vi "CLD 16 state machine front panel.vi"() -> ()   [LabVIEW 2019]
doc: "CLD 16 Exercise"
uses:
  CLD 16 Control Panel.ctl
  CLD 16 Status Panel.ctl
  CLD 16 state enum.ctl
panel:
  out "error out":errorcluster
  in  "error in (no error)":errorcluster
  in  "Stop Button":bool
  out "Line Two Active":bool
  out "Line One Active":bool
  in  "Control Panel Two":T1 {"Tons of Peanuts" scale=0.0..10.0}
  out "Process Control":T2 {"Process Value" format="%#.3g"}
  in  "Control Panel One":T1 {"Tons of Peanuts" scale=0.0..10.0}
  # "Display Panel"
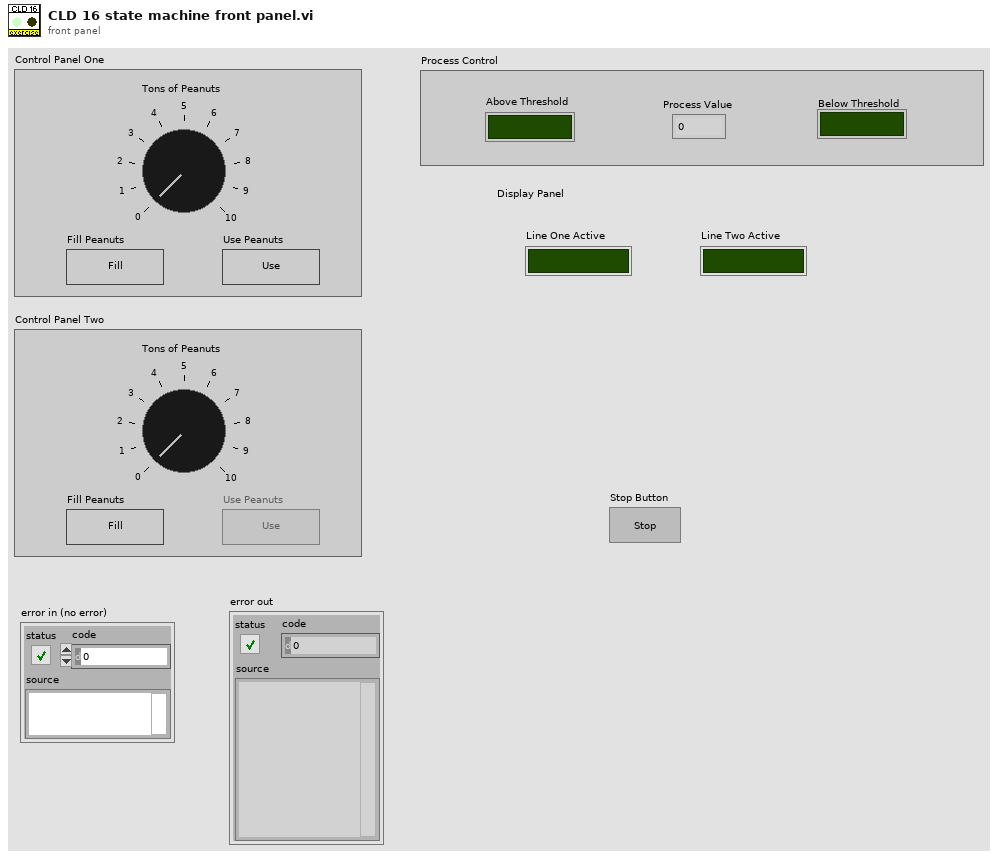
[diagram p1: front panel]
types:
  T1 = typedef "CLD 16 Control Panel.ctl" = cluster{"Tons of Peanuts":i8, "Fill Peanuts":bool, "Use Peanuts":bool}
  T2 = typedef "CLD 16 Status Panel.ctl" = cluster{"Above Threshold":bool, "Below Threshold":bool, "Process Value":dbl}
  T3 = typedef "CLD 16 state enum.ctl" = enum16{"initialize", "use", "idle"}
  T4 = enum8{"Enabled", "Disabled", "Disabled and Grayed Out"}
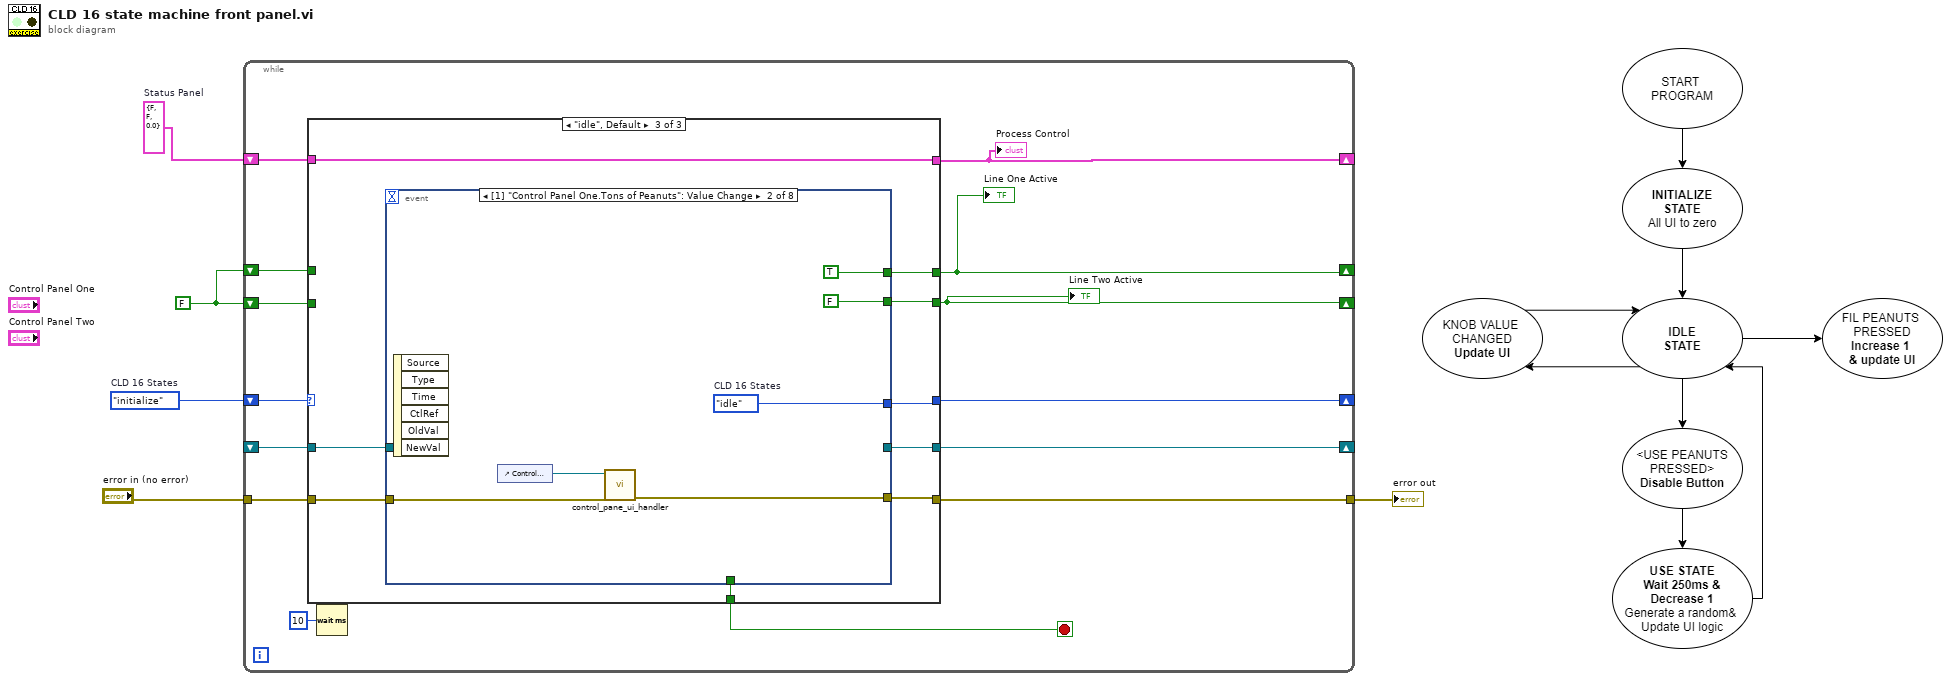
[diagram p0: block diagram]
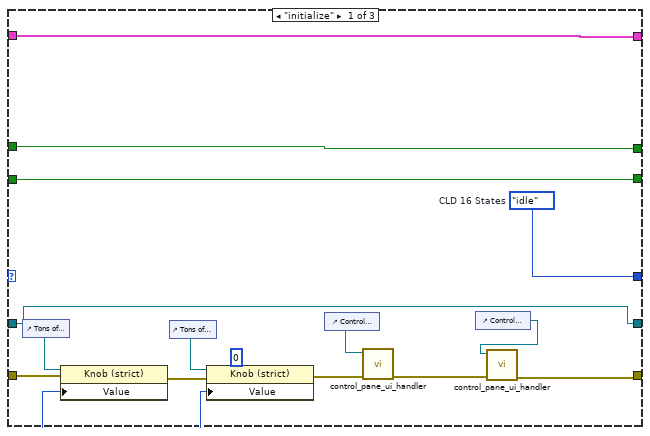
[diagram p2: hidden frame]
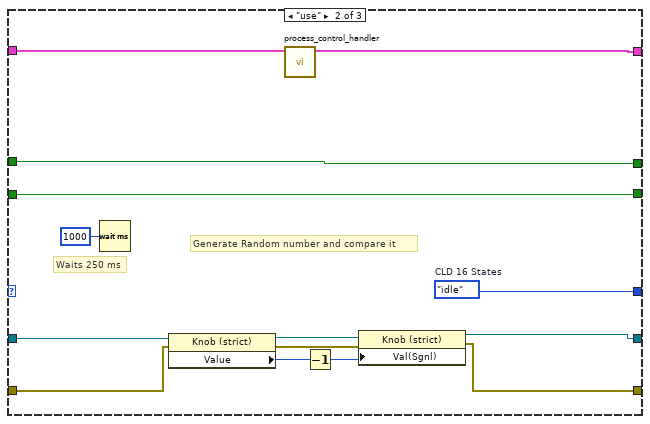
[diagram p3: hidden frame]
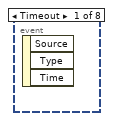
[diagram p4: hidden frame]
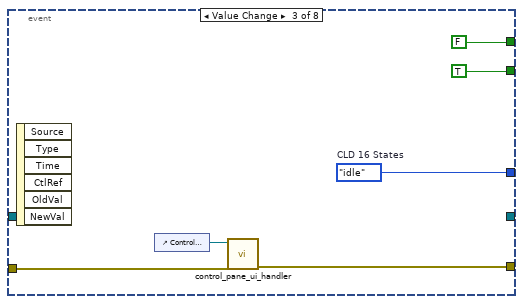
[diagram p5: hidden frame]
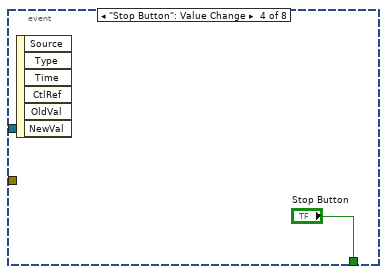
[diagram p6: hidden frame]
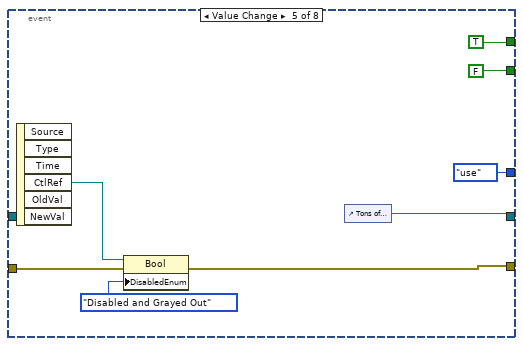
[diagram p7: hidden frame]
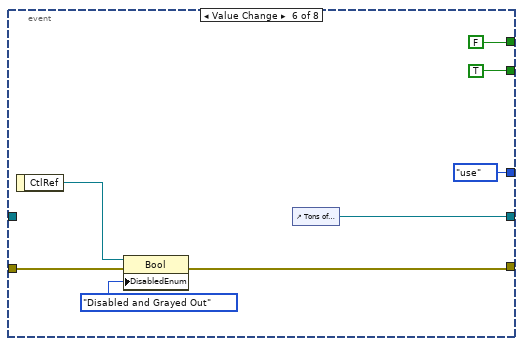
[diagram p8: hidden frame]
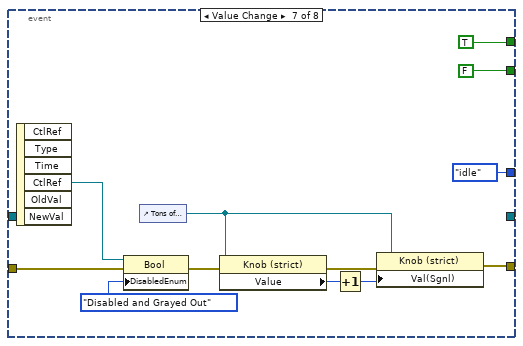
[diagram p9: hidden frame]
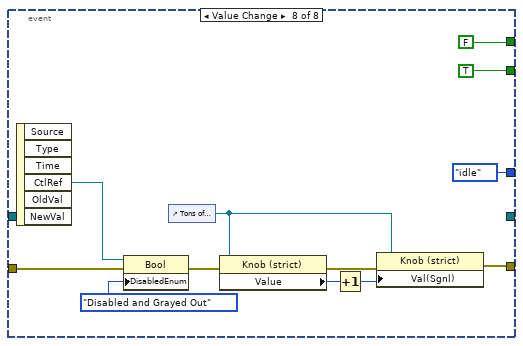
[diagram p10: hidden frame]
diagram:
  w1 = FALSE ("Line Two Active")
  w2 = T2 {"Above Threshold"=FALSE, "Below Threshold"=FALSE, "Process Value"=0.0}  # Status Panel
  w5 = CLD_16_state_enum."initialize"  # CLD 16 States
  n1 = while {
    shift-right: [w18] -> _
    shift-left: w5 -> [w19]
    tunnel: "error in (no error)" -> [w17]
    tunnel: [w16] -> w3
    shift-right: [w14] -> _
    shift-left: w2 -> [w13]
    shift-right: [w9] -> _
    shift-left: w1 -> [w12]
    shift-right: [w10] -> _
    shift-left: w1 -> [w11]
    shift-right: [w8] -> _
    shift-left: _ -> [w7]
    stop <- w6 stop-if-true
    n2 = case shown="\"idle\", Default" w19 {
      tunnel: [w23 w36 w54] -> w14
      tunnel: [w34 w48 w55] -> w18
      tunnel: w17 -> [w31 w44 w57]
      tunnel: [w25 w38 w56] -> w16
      tunnel: w13 -> [w23 w37 w54]
      tunnel: [w22 w46 w53] -> w9
      tunnel: w12 -> [w22 w46 _]
      tunnel: [w21 w45 w52] -> w10
      tunnel: w11 -> [w21 w45 _]
      tunnel: [w20 w35 w51] -> w8
      tunnel: w7 -> [w20 w43 w50]
      tunnel: [_ _ w49] -> w6
      frame "initialize" {
        w29 = i8 0 ("Value")
        w34 = CLD_16_state_enum."idle"  # CLD 16 States
        n3 = control-ref of="Tons of Peanuts"() -> (w32:refnum<vi>)
        n4 = property class="Knob (strict)"(reference=w32, error in=w31, "Value"=w29) -> (error out=w30:errorcluster)  [unwired: 1 out]
        n5 = control-ref of="Tons of Peanuts"() -> (w33:refnum<vi>)
        n6 = property class="Knob (strict)"(reference=w33, error in=w30, "Value"=w29) -> (error out=w27:errorcluster)  [unwired: 1 out]
        n7 = control-ref of="Control Panel One"() -> (w28:refnum<vi>)
        n8 = call "control_pane_ui_handler.vi"("error in (no error)"=w27, "Control Panel In"=w28) -> ("error out"=w26:errorcluster)  [unwired: 9 in]
        n9 = control-ref of="Control Panel Two"() -> (w24:refnum<vi>)
        n10 = call "control_pane_ui_handler.vi"("error in (no error)"=w26, "Control Panel In"=w24) -> ("error out"=w25:errorcluster)  [unwired: 9 in]
      }
      frame "use" {
        w48 = CLD_16_state_enum."idle"  # CLD 16 States
        # "Generate Random number and compare it"
        # "Waits 250 ms"
        n11 = Wait (ms)(milliseconds to wait=u32 1000) -> ()  [unwired: 1 out]
        n12 = property class="Knob (strict)"(reference=w43, error in=w44) -> (reference out=w42:refnum<vi>, error out=w41:errorcluster, "Value"=w40:i8)
        n13 = call "process_control_handler.vi"("Status Panel in"=w37) -> ("Status Panel out"=w36:T2)  [unwired: 10 in]
        n14 = Decrement(x=w40) -> (x-1=w39:i8)
        n15 = property class="Knob (strict)"(reference=w42, error in=w41, "Val(Sgnl)"=w39) -> (reference out=w35:refnum<vi>, error out=w38:errorcluster)
      }
      frame "idle", Default {
        n16 = event shown="[1] \"Control Panel One.Tons of Peanuts\": Value Change" {
          selector: _ -> [_ _ _ _ _ _ _ _]
          dyn-events: _ -> [_ _ _ _ _ _ _ _]
          timeout: _ -> [_ _ _ _ _ _ _ _]
          tunnel: w57 -> [_ w63 w69 _ w77 w85 w97 w109]
          tunnel: [_ w62 w68 _ w72 w80 w94 w105] -> w56
          tunnel: [_ w60 w66 _ CLD_16_state_enum."use" ("CLD 16 States") CLD_16_state_enum."use" ("CLD 16 States") CLD_16_state_enum."idle" ("CLD 16 States") CLD_16_state_enum."idle" ("CLD 16 States")] -> w55
          tunnel: [_ TRUE ("Line Two Active") FALSE ("Line Two Active") _ TRUE ("Line Two Active") FALSE ("Line Two Active") TRUE ("Line Two Active") FALSE ("Line Two Active")] -> w53
          tunnel: [_ FALSE ("Line Two Active") TRUE ("Line Two Active") _ FALSE ("Line Two Active") TRUE ("Line Two Active") FALSE ("Line Two Active") TRUE ("Line Two Active")] -> w52
          tunnel: [_ _ _ _ w71 w79 _ _] -> w51
          tunnel: w50 -> [_ _ _ _ _ _ _ _]
          tunnel: [_ _ _ "Stop Button" _ _ _ _] -> w49
          event Timeout {
            n17 = event-data() -> ()  [unwired: 1 in, 3 out]
          }
          event Value Change {
            w60 = CLD_16_state_enum."idle"  # CLD 16 States
            n18 = event-data() -> ()  [unwired: 1 in, 6 out]
            n19 = control-ref of="Control Panel One"() -> (w61:refnum<vi>)
            n20 = call "control_pane_ui_handler.vi"("error in (no error)"=w63, "Control Panel In"=w61) -> ("error out"=w62:errorcluster)  [unwired: 9 in]
          }
          event Value Change {
            w66 = CLD_16_state_enum."idle"  # CLD 16 States
            n21 = event-data() -> ()  [unwired: 1 in, 6 out]
            n22 = control-ref of="Control Panel Two"() -> (w67:refnum<vi>)
            n23 = call "control_pane_ui_handler.vi"("error in (no error)"=w69, "Control Panel In"=w67) -> ("error out"=w68:errorcluster)  [unwired: 9 in]
          }
          event "Stop Button": Value Change {
            n24 = event-data() -> ()  [unwired: 1 in, 6 out]
          }
          event Value Change {
            n25 = event-data() -> ("CtlRef"=w78:refnum<vi>)  [unwired: 1 in, 5 out]
            n26 = property class="Bool"(reference=w78, error in=w77, "DisabledEnum"=T4."Disabled and Grayed Out" ("Disabled")) -> (error out=w72:errorcluster)  [unwired: 1 out]
            n27 = control-ref of="Tons of Peanuts"() -> (w71:refnum<vi>)
          }
          event Value Change {
            n28 = event-data() -> ("CtlRef"=w86:refnum<vi>)  [unwired: 1 in]
            n29 = property class="Bool"(reference=w86, error in=w85, "DisabledEnum"=T4."Disabled and Grayed Out" ("Disabled")) -> (error out=w80:errorcluster)  [unwired: 1 out]
            n30 = control-ref of="Tons of Peanuts"() -> (w79:refnum<vi>)
          }
          event Value Change {
            n31 = event-data() -> ("CtlRef"=w98:refnum<vi>)  [unwired: 1 in, 5 out]
            n32 = property class="Bool"(reference=w98, error in=w97, "DisabledEnum"=T4."Disabled and Grayed Out" ("Disabled")) -> (error out=w95:errorcluster)  [unwired: 1 out]
            n33 = control-ref of="Tons of Peanuts"() -> (w87:refnum<vi>)
            n34 = property class="Knob (strict)"(reference=w87, error in=w95) -> (error out=w92:errorcluster, "Value"=w91:i8)  [unwired: 1 out]
            n35 = Increment(x=w91) -> (x+1=w90:i8)
            n36 = property class="Knob (strict)"(reference=w87, error in=w92, "Val(Sgnl)"=w90) -> (error out=w94:errorcluster)  [unwired: 1 out]
          }
          event Value Change {
            n37 = event-data() -> ("CtlRef"=w110:refnum<vi>)  [unwired: 1 in, 5 out]
            n38 = property class="Bool"(reference=w110, error in=w109, "DisabledEnum"=T4."Disabled and Grayed Out" ("Disabled")) -> (error out=w107:errorcluster)  [unwired: 1 out]
            n39 = control-ref of="Tons of Peanuts"() -> (w106:refnum<vi>)
            n40 = property class="Knob (strict)"(reference=w106, error in=w107) -> (error out=w103:errorcluster, "Value"=w102:i8)  [unwired: 1 out]
            n41 = Increment(x=w102) -> (x+1=w101:i8)
            n42 = property class="Knob (strict)"(reference=w106, error in=w103, "Val(Sgnl)"=w101) -> (error out=w105:errorcluster)  [unwired: 1 out]
          }
        }
      }
    }
    "Process Control" <- w14
    "Line Two Active" <- w10
    "Line One Active" <- w9
    n43 = Wait (ms)(milliseconds to wait=u32 10) -> ()  [unwired: 1 out]
  }
  "error out" <- w3
